vi "test_trigger.vi"() -> ()   [LabVIEW 2016, in "_Delay Line.lvlib" / "DAQmx Delay Line.lvclass"]
uses:
  DAQmx Delay Line.lvclass
  Drivers/C8855-01/Trigger Mode.ctl
  Drivers/C8855-01/Transfer Mode.ctl
  <vilib>/DAQmx/create/channels.llb/DAQmx Create Channel (CO-Pulse Generation-Time).vi
  <vilib>/DAQmx/configure/timing.llb/DAQmx Timing (Implicit).vi
  Drivers/C8855-01/C8855-01.lvlib
panel:
  out "Data":i32[](graph)
  in  "Initial Delay (s)":dbl=5.0 format="%#_13g"
  out "Photon Counter ID":u8
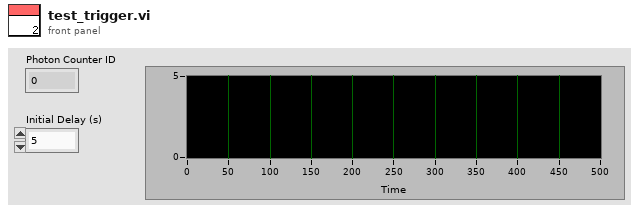
[diagram p1: front panel]
types:
  T1 = typedef "Drivers.lvlib/C8855-01.lvlib/Transfer Mode.ctl" = u8
  T2 = typedef "Drivers.lvlib/C8855-01.lvlib/Trigger Mode.ctl" = u8
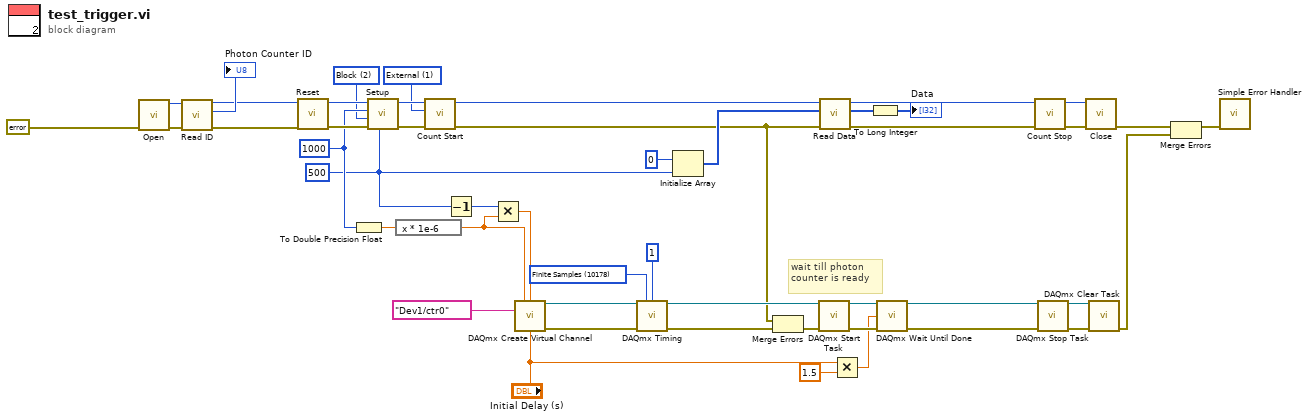
[diagram p0: block diagram]
diagram:
  w14 = T1 2 items=["Single"=1, "Block"=2] ("Transfer Mode")
  w22 = 10178 items=["Finite Samples"=10178, "Continuous Samples"=10123, "Hardware Timed Single Point"=12522] ("sample mode")
  w21 = 500 ("Number of Gate")
  w29 = u32 1000 ("Gate Time (us)")
  w38 = T2 1 items=["Software", "External"] ("Trigger Mode")
  # "wait till photon counter is ready"
  n1 = call "Open.vi"("error in (no error)"=errorcluster {"status"=FALSE, "code"=0, "source"=""}) -> ("error out"=w46:errorcluster, "Handle"=w47:u32)  [unwired: 9 in]
  n2 = call "Read ID.vi"("error in (no error)"=w46, "handle in"=w47) -> ("error out"=w44:errorcluster, "ID"=→"Photon Counter ID":u8, "handle out"=w43:u32)  [unwired: 7 in]
  n3 = call "Reset.vi"("error in (no error)"=w44, "handle in"=w43) -> ("error out"=w42:errorcluster, "handle out"=w39:u32)  [unwired: 8 in]
  n4 = To Double Precision Float(number=w29) -> (double precision float=w28:dbl)
  n5 = call "Setup.vi"("Number of Gate"=w21, "error in (no error)"=w42, "Transfer Mode"=w14, "Gate Time (us)"=w29, "Handle"=w39) -> ("error out"=w41:errorcluster, "Handle out"=w40:u32)  [unwired: 5 in]
  n6 = expression code="x * 1e-6"(w28) -> (w23:dbl)
  n7 = call "Count Start.vi"("error in (no error)"=w41, "Trigger Mode"=w38, "handle in"=w40) -> ("error out"=w4:errorcluster, "handle out"=w36:u32)  [unwired: 7 in]
  n8 = Decrement(x=w21) -> (x-1=w27:i32)
  n9 = Multiply(x=w27, y=w23) -> (x*y=w26:dbl)
  n10 = call-poly <vilib>:"DAQmx Create Virtual Channel.vi"("high time"=w23, "low time"=w26, "counter"=tag "Dev1/ctr0" ("physical channels"), "initial delay"="Initial Delay (s)") -> ("task out"=w25:refnum<k21>, "error out"=w24:errorcluster)  [unwired: 10 in]
  n11 = call-poly <vilib>:"DAQmx Timing.vi"("task/channels in"=w25, "sample mode"=w22, "samples per channel"=1, "error in"=w24) -> ("task out"=w20:refnum<k21>, "error out"=w6:errorcluster)  [unwired: 10 in]
  n12 = Initialize Array(u16 0 ("element"), w21) -> (w34:u16[])
  n13 = Merge Errors(w4, w6) -> (w5:errorcluster)
  n14 = call <vilib>:"DAQmx Start Task.vi"("task/channels in"=w20, "error in"=w5) -> ("task out"=w19:refnum<k21>, "error out"=w18:errorcluster)  [unwired: 12 in]
  n15 = call "Read Data.vi"("error in (no error)"=w4, "buffer in"=w34, "handle in"=w36) -> ("error out"=w12:errorcluster, "buffer out"=w35:u16[], "handle out"=w33:u32)  [unwired: 6 in]
  n16 = Multiply(x="Initial Delay (s)", y=1.5) -> (x*y=w1:dbl)
  n17 = To Long Integer(number=w35) -> (32bit integer=→"Data":i32[])
  n18 = call <vilib>:"DAQmx Wait Until Done.vi"("task/channels in"=w19, "timeout (sec)"=w1, "error in"=w18) -> ("task out"=w9:refnum<k21>, "error out"=w11:errorcluster)  [unwired: 11 in]
  n19 = call "Count Stop.vi"("error in (no error)"=w12, "handle in"=w33) -> ("error out"=w31:errorcluster, "handle out"=w32:u32)  [unwired: 8 in]
  n20 = call <vilib>:"DAQmx Stop Task.vi"("task/channels in"=w9, "error in"=w11) -> ("task out"=w8:refnum<k21>, "error out"=w10:errorcluster)  [unwired: 12 in]
  n21 = call "Close.vi"("error in (no error)"=w31, "handle in"=w32) -> ("error out"=w17:errorcluster)  [unwired: 9 in]
  n22 = call <vilib>:"DAQmx Clear Task.vi"("task in"=w8, "error in"=w10) -> ("error out"=w15:errorcluster)  [unwired: 13 in]
  n23 = Merge Errors(w17, w15) -> (w16:errorcluster)
  n24 = call <vilib>:"Simple Error Handler.vi"("error in (no error)"=w16) -> ()  [unwired: 4 in, 5 out]
